vi "tempconfigtiff.vi"(1 "Temp Config in":T1, 2 "command":string) -> (0 "Temp Config out":T1)   [LabVIEW 2010]
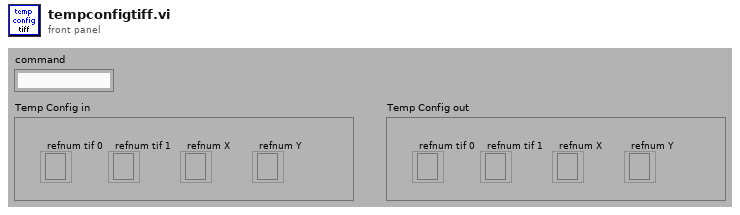
[diagram p1: front panel]
types:
  T1 = cluster{"refnum tif 0":refnum<file>, "refnum tif 1":refnum<file>, "refnum X":refnum<file>, "refnum Y":refnum<file>}
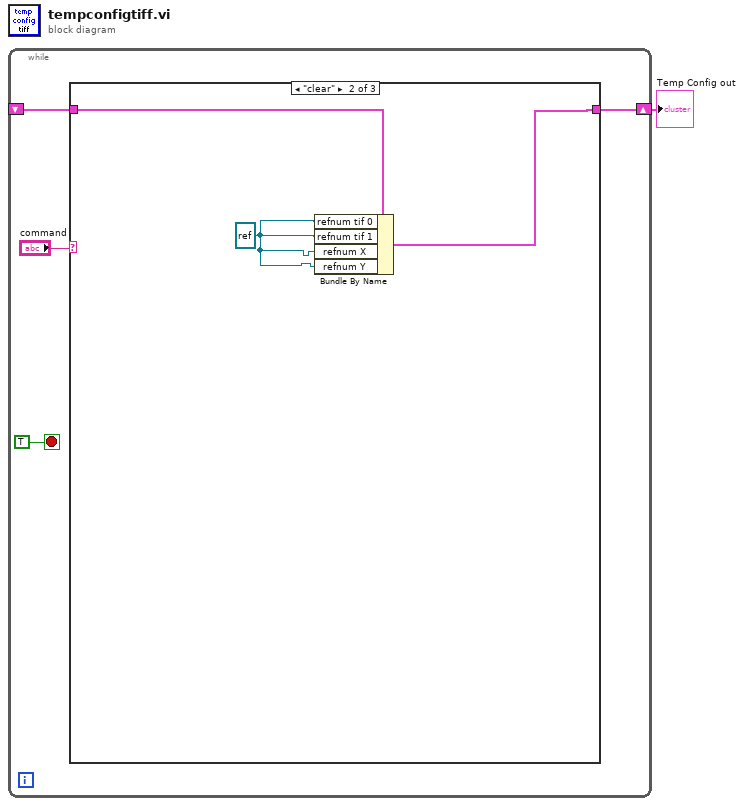
[diagram p0: block diagram]
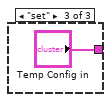
[diagram p3: hidden frame]
diagram:
  n1 = while {
    shift-right: [w3] -> w1
    shift-left: _ -> [w2]
    stop <- TRUE stop-if-true
    n2 = case shown="\"clear\"" "command" {
      tunnel: [w6 w7 "Temp Config in"] -> w3
      tunnel: w2 -> [w6 w9 _]
      frame "get", Default {
      }
      frame "clear" {
        w8 = refnum<file> refnum ("refnum tif 1")
        n3 = Bundle By Name(cluster=w9, "refnum tif 0"=w8, "refnum tif 1"=w8, "refnum X"=w8, "refnum Y"=w8) -> (w7:T1)
      }
      frame "set" {
      }
    }
  }
  "Temp Config out" <- w1
